vi "Test Assertion Report Ordering.vi"(8 "error in (no error)":errorcluster) -> (0 "error out":errorcluster)   [LabVIEW 2020]
uses:
  classes/Test/Test.lvclass
  classes/Assert/Assert.lvclass
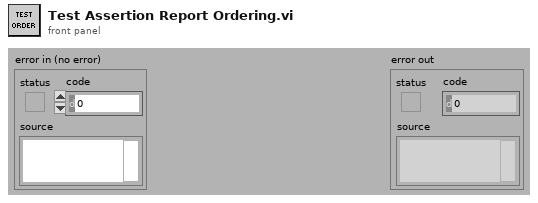
[diagram p1: front panel]
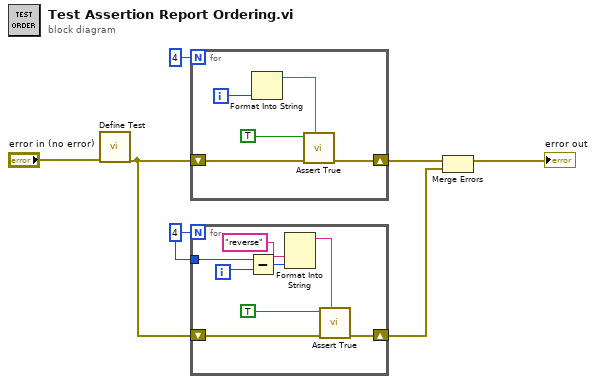
[diagram p0: block diagram]
diagram:
  w4 = 4
  n1 = call "Define Test.vi"("error in (no error)"="error in (no error)") -> ("error out"=w5:errorcluster)  [unwired: 9 in, 1 out]
  n2 = for {
    N: 4 -> [_]
    shift-right: [w11] -> w2
    shift-left: w5 -> [w12]
    i -> [w9]
    n3 = Format Into String(w9) -> (resulting string=w8:string)  [unwired: 3 in, 1 out]
    n4 = call "Assert True.vi"("Label"=w8, "error in (no error)"=w12, "True?"=TRUE) -> ("error out"=w11:errorcluster)  [unwired: 7 in, 1 out]
  }
  n5 = for {
    N: w4 -> [_]
    shift-right: [w19] -> w3
    shift-left: w5 -> [w20]
    tunnel: w4 -> [w17]
    i -> [w16]
    n6 = Subtract(x=w17, y=w16) -> (x-y=w15:i32)
    n7 = Format Into String("reverse", w15) -> (resulting string=w14:string)  [unwired: 3 in, 1 out]
    n8 = call "Assert True.vi"("Label"=w14, "error in (no error)"=w20, "True?"=TRUE) -> ("error out"=w19:errorcluster)  [unwired: 7 in, 1 out]
  }
  n9 = Merge Errors(w2, w3) -> (→"error out":errorcluster)
